vi "JoystickSimulator.vi"() -> ()   [LabVIEW 2016]
doc: "This is a stand alone VI not intended for robot code. This VI outputs Joystick values based on the mouse positon on the front pannel. A gauge is provided to allow the user to visuialize the input and the circular range a joystick limits the user to.\n\nCreated by Team 4130 for use in the 2016-2017 FRC season"
uses:
  <vilib>/Rock Robotics/Network Tables/NT Read Number.vi
  <vilib>/Rock Robotics/Network Tables/NT Write Numeric Array.vi
  <vilib>/Rock Robotics/Network Tables/NT Write Boolean.vi
panel:
  out "Reverse":bool=TRUE
  out "?":dbl(knob) scale=-180.0..180.0
  # "Click the dial to reverse\nthis simulates pushing down\non the joystick"
  # "Moving the mouse across the dial simulates\na joystick"
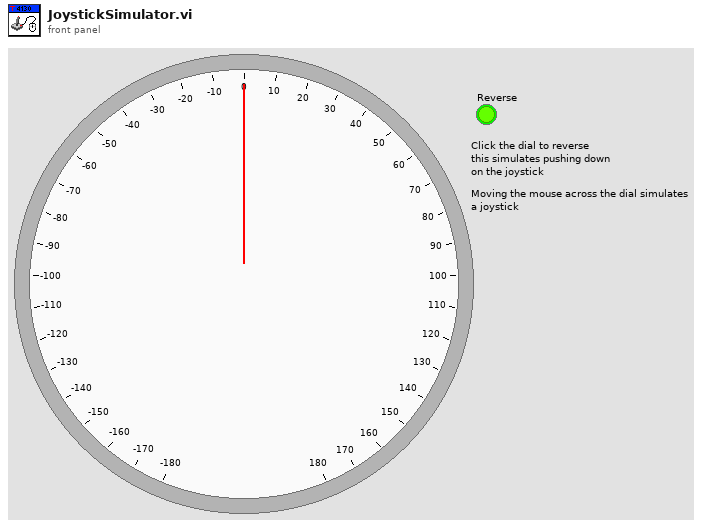
[diagram p1: front panel]
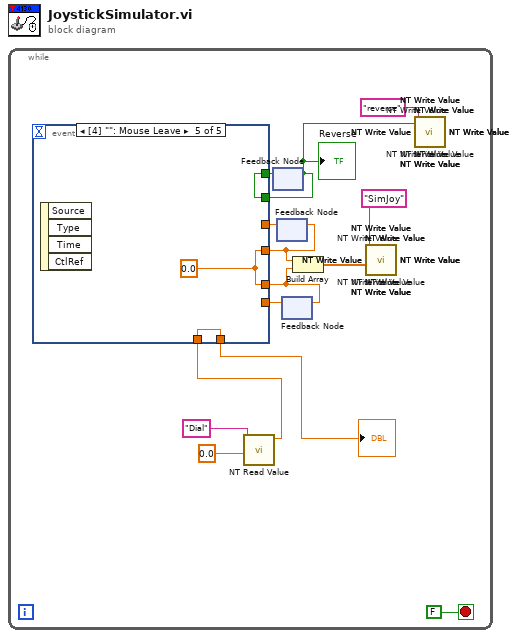
[diagram p0: block diagram]
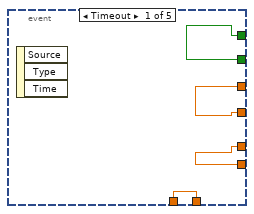
[diagram p2: hidden frame]
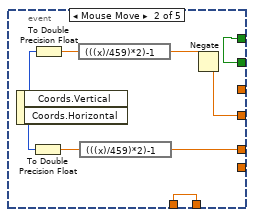
[diagram p3: hidden frame]
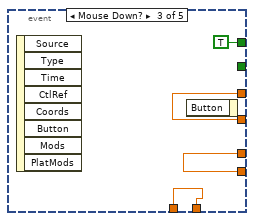
[diagram p4: hidden frame]
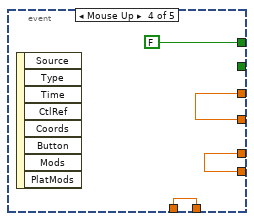
[diagram p5: hidden frame]
diagram:
  n1 = while {
    stop <- FALSE stop-if-true
    n2 = call-poly <vilib>:"NT Read Value.vi"("Default Value"=0.0, "Name"="Dial") -> ("Numeric"=w2:dbl)  [unwired: 8 in, 1 out]
    n3 = feedback #1() -> (w8:bool)  [unwired: 1 in]
    "Reverse" <- w8
    n4 = feedback #2() -> (w5:dbl)  [unwired: 1 in]
    n5 = feedback #3() -> (w3:dbl)  [unwired: 1 in]
    n6 = event shown="[4] \"\": Mouse Leave" {
      selector: _ -> [_ _ _ _ _]
      dyn-events: _ -> [_ _ _ _ _]
      timeout: _ -> [_ _ _ _ _]
      tunnel: [w17 w21 w30 w34 w37] -> w6
      tunnel: [w16 w22 w29 w33 w37] -> w4
      tunnel: [w18 w20 TRUE FALSE w38] -> w9
      tunnel: w8 -> [w18 w20 _ _ w38]
      tunnel: w5 -> [w17 _ w30 w34 _]
      tunnel: w3 -> [w16 _ w29 w33 _]
      tunnel: w2 -> [w15 w19 w28 w32 w36]
      tunnel: [w15 w19 w28 w32 w36] -> w1
      event Timeout {
        n7 = event-data() -> ()  [unwired: 1 in, 3 out]
      }
      event Mouse Move {
        n8 = event-data() -> ("Coords.Vertical"=w25:i32, "Coords.Horizontal"=w26:i32)  [unwired: 1 in]
        n9 = To Double Precision Float(number=w26) -> (double precision float=w23:dbl)
        n10 = To Double Precision Float(number=w25) -> (double precision float=w24:dbl)
        n11 = expression code="(((x)/459)*2)-1"(w24) -> (w27:dbl)
        n12 = expression code="(((x)/459)*2)-1"(w23) -> (w22:dbl)
        n13 = Negate(x=w27) -> (-x=w21:dbl)
      }
      event Mouse Down? {
        n14 = event-data() -> ()  [unwired: 1 in, 8 out]
        n15 = event-data() -> ()  [unwired: 2 in, 1 out]
      }
      event Mouse Up {
        n16 = event-data() -> ()  [unwired: 1 in, 8 out]
      }
      event Mouse Leave {
        w37 = 0.0
        n17 = event-data() -> ()  [unwired: 1 in, 4 out]
      }
    }
    "?" <- w1
    n18 = feedback-in #1(w9) -> ()
    n19 = feedback-in #2(w6) -> ()
    n20 = feedback-in #3(w4) -> ()
    n21 = Build Array(w6, w4) -> (w14:dbl[])
    n22 = call-poly <vilib>:"NT Write Value.vi"() -> ()  [unwired: 11 in, 1 out]
    n23 = call-poly <vilib>:"NT Write Value.vi"() -> ()  [unwired: 11 in, 1 out]
    n24 = call-poly <vilib>:"NT Write Value.vi"() -> ()  [unwired: 11 in, 1 out]
    n25 = call-poly <vilib>:"NT Write Value.vi"() -> ()  [unwired: 11 in, 1 out]
    n26 = call-poly <vilib>:"NT Write Value.vi"() -> ()  [unwired: 11 in, 1 out]
    n27 = call-poly <vilib>:"NT Write Value.vi"() -> ()  [unwired: 11 in, 1 out]
    n28 = call-poly <vilib>:"NT Write Value.vi"() -> ()  [unwired: 11 in, 1 out]
    n29 = call-poly <vilib>:"NT Write Value.vi"() -> ()  [unwired: 11 in, 1 out]
    n30 = call-poly <vilib>:"NT Write Value.vi"() -> ()  [unwired: 11 in, 1 out]
    n31 = call-poly <vilib>:"NT Write Value.vi"() -> ()  [unwired: 11 in, 1 out]
    n32 = call-poly <vilib>:"NT Write Value.vi"() -> ()  [unwired: 11 in, 1 out]
    n33 = call-poly <vilib>:"NT Write Value.vi"() -> ()  [unwired: 11 in, 1 out]
    n34 = call-poly <vilib>:"NT Write Value.vi"() -> ()  [unwired: 11 in, 1 out]
    n35 = call-poly <vilib>:"NT Write Value.vi"() -> ()  [unwired: 11 in, 1 out]
    n36 = call-poly <vilib>:"NT Write Value.vi"() -> ()  [unwired: 11 in, 1 out]
    n37 = call-poly <vilib>:"NT Write Value.vi"("Numeric Array"=w14, "Name"="SimJoy") -> ()  [unwired: 9 in, 1 out]
    n38 = call-poly <vilib>:"NT Write Value.vi"("Boolean"=w8, "Name"="reverse") -> ()  [unwired: 9 in, 1 out]
    n39 = call-poly <vilib>:"NT Write Value.vi"() -> ()  [unwired: 11 in, 1 out]
    n40 = call-poly <vilib>:"NT Write Value.vi"() -> ()  [unwired: 11 in, 1 out]
    n41 = call-poly <vilib>:"NT Write Value.vi"() -> ()  [unwired: 11 in, 1 out]
    n42 = call-poly <vilib>:"NT Write Value.vi"() -> ()  [unwired: 11 in, 1 out]
    n43 = call-poly <vilib>:"NT Write Value.vi"() -> ()  [unwired: 11 in, 1 out]
    n44 = call-poly <vilib>:"NT Write Value.vi"() -> ()  [unwired: 11 in, 1 out]
    n45 = call-poly <vilib>:"NT Write Value.vi"() -> ()  [unwired: 11 in, 1 out]
    n46 = call-poly <vilib>:"NT Write Value.vi"() -> ()  [unwired: 11 in, 1 out]
    n47 = call-poly <vilib>:"NT Write Value.vi"() -> ()  [unwired: 11 in, 1 out]
    n48 = call-poly <vilib>:"NT Write Value.vi"() -> ()  [unwired: 11 in, 1 out]
    n49 = call-poly <vilib>:"NT Write Value.vi"() -> ()  [unwired: 11 in, 1 out]
    n50 = call-poly <vilib>:"NT Write Value.vi"() -> ()  [unwired: 11 in, 1 out]
    n51 = call-poly <vilib>:"NT Write Value.vi"() -> ()  [unwired: 11 in, 1 out]
    n52 = call-poly <vilib>:"NT Write Value.vi"() -> ()  [unwired: 11 in, 1 out]
    n53 = call-poly <vilib>:"NT Write Value.vi"() -> ()  [unwired: 11 in, 1 out]
  }
